vi "GetEventFrameInformation.vi"(8 "error in (no error)":errorcluster, 11 "Device Ref in":T3 format="%.0x") -> (0 "error out":errorcluster, 2 "EventFrames":T1[](array[typedef]) {"Channel Data Ref" format="%.0x"}, 3 "Device Ref out":T3 format="%.0x")   [LabVIEW 2020, in "FlexRay Custom Device Engine.lvlib"]
uses:
  FlexRay Custom Device Engine.lvlib
  <vilib>/NI VeriStand/Custom Device API/Custom Device Item Ref.ctl
  Shared/FREventInfo.ctl
  <vilib>/NI VeriStand/Custom Device API/Data Reference.ctl
  <vilib>/NI VeriStand/Custom Device API/Data Access Type.ctl
  Shared/Constants.vi
  <vilib>/NI VeriStand/Custom Device API/Get Item Property (Variant).vi
  <vilib>/NI VeriStand/Custom Device API/Custom Device API.lvlib
  <vilib>/NI VeriStand/Custom Device Tools/Custom Device Utility Library/Custom Device Utility Library.lvlib
  Shared/FlexRay Custom Device Shared.lvlib
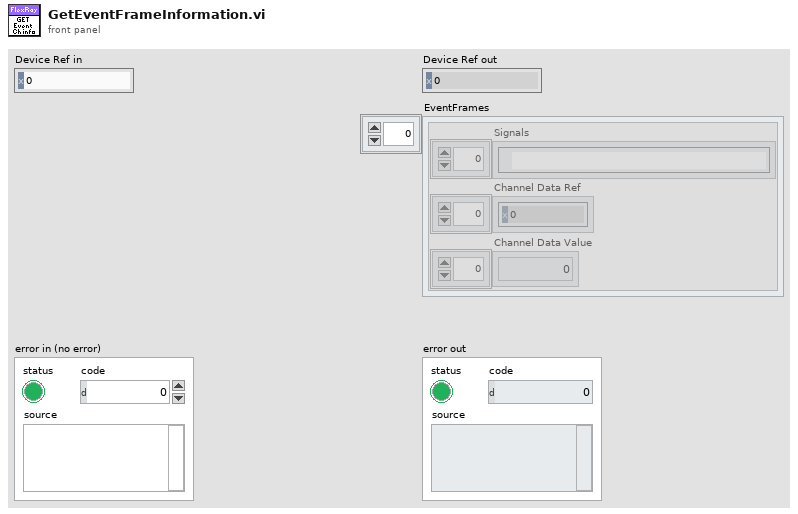
[diagram p1: front panel]
types:
  T1 = typedef "FlexRay Custom Device Shared.lvlib/FREventInfo.ctl" = cluster{"Signals":refnum<k21>[], "Channel Data Ref":T2[], "Channel Data Value":dbl[]}
  T2 = typedef "Custom Device API.lvlib/Data Reference.ctl" = i32
  T3 = typedef "Custom Device API.lvlib/Custom Device Item Ref.ctl" = u64
  T4 = typedef "Custom Device API.lvlib/Data Access Type.ctl" = enum16{"Read", "Write"}
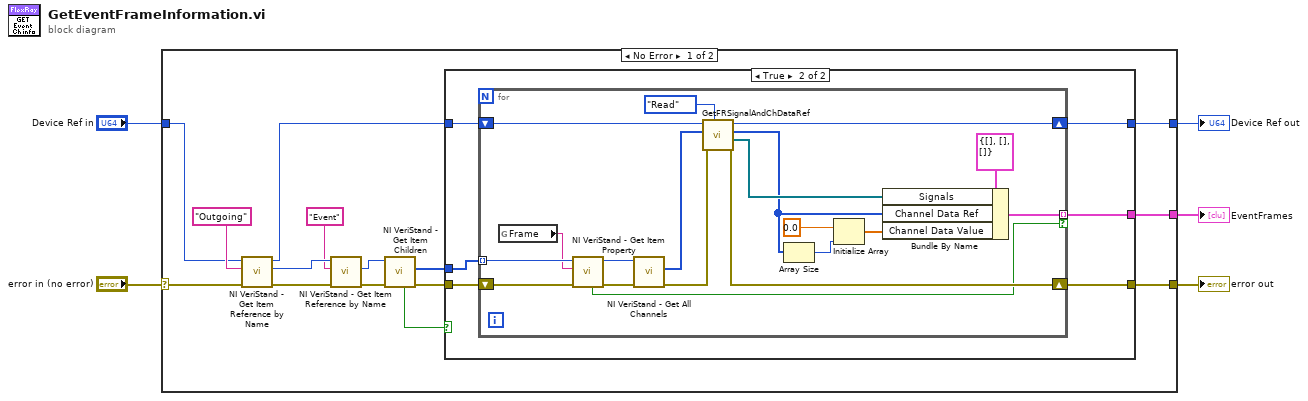
[diagram p0: block diagram]
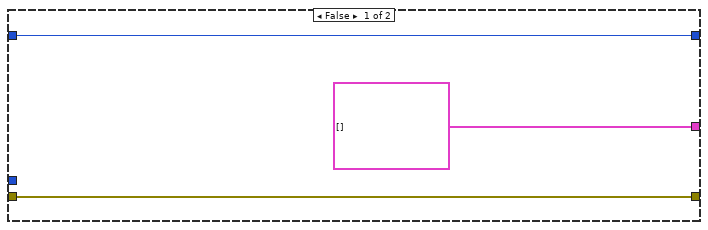
[diagram p2: hidden frame]
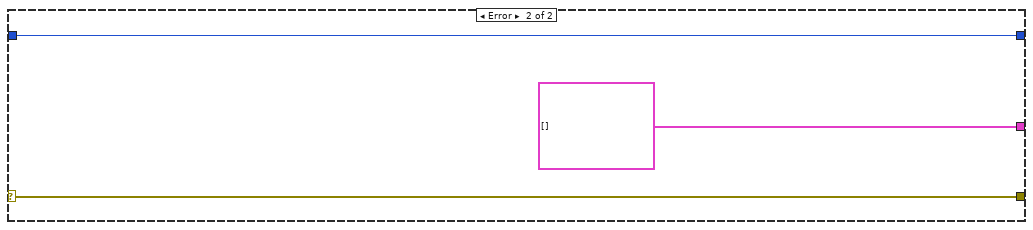
[diagram p3: hidden frame]
diagram:
  n1 = case shown="No Error" "error in (no error)" {
    selector: "error in (no error)" -> [w9 w50]
    tunnel: [w20 w50] -> w5
    tunnel: [w19 w51] -> w4
    tunnel: "Device Ref in" -> [w16 w51]
    tunnel: [w6 T1[] []] -> w1
    frame No Error {
      n2 = call <vilib>:"NI VeriStand - Get Item Reference by Name.vi"("error in (no error)"=w9, "Item Name"="Outgoing" ("Section Name"), "Parent Ref in"=w16) -> ("error out"=w15:errorcluster, "Item Ref"=w14:T3, "Parent Ref out"=w7:T3)  [unwired: 5 in, 1 out]
      n3 = call <vilib>:"NI VeriStand - Get Item Reference by Name.vi"("error in (no error)"=w15, "Item Name"="Event", "Parent Ref in"=w14) -> ("error out"=w13:errorcluster, "Item Ref"=w11:T3)  [unwired: 5 in, 2 out]
      n4 = call <vilib>:"NI VeriStand - Get Item Children.vi"("error in (no error)"=w13, "Item Ref in"=w11) -> ("error out"=w8:errorcluster, "Child Refs"=w18:T3[], "Found"=w10:bool)  [unwired: 6 in, 1 out]
      n5 = case shown="True" w10 {
        tunnel: w7 -> [w22 w29]
        tunnel: [w22 w28] -> w19
        tunnel: w8 -> [w23 w27]
        tunnel: [w23 w26] -> w20
        tunnel: w18 -> [_ w25]
        tunnel: [T1[] [] w24] -> w6
        frame False {
        }
        frame True {
          n6 = for {
            shift-right: [w43] -> w28
            shift-left: w29 -> [w46]
            shift-right: [w41] -> w26
            shift-left: w27 -> [w31]
            tunnel: w25 -> [w48] mode=indexing
            tunnel: [w38] -> w24 mode=indexing if=w33
            n7 = global read "Constants.vi" "Frame"() -> (w47:string)
            n8 = call-poly <vilib>:"NI VeriStand - Get Item Property.vi"("error in (no error)"=w31, "Property Name"=w47, "Item Ref in"=w48) -> ("error out"=w30:errorcluster, "Item Ref out"=w32:T3, "Found?"=w33:bool)  [unwired: 5 in, 1 out]
            n9 = call <vilib>:"NI VeriStand - Get All Channels.vi"("error in"=w30, "Section Ref in"=w32) -> ("error out"=w44:errorcluster, "Channel Refs"=w45:T3[])  [unwired: 6 in, 2 out]
            n10 = call "GetFRSignalAndChDataRef.vi"("Access"=Data_Access_Type."Read", "error in (no error)"=w44, "Channel Refs"=w45, "Device Ref in"=w46) -> ("error out"=w41:errorcluster, "FR Signals"=w39:refnum<k21>[], "Channel Data Ref"=w37:T2[], "Device Ref out"=w43:T3)  [unwired: 4 in]
            n11 = Array Size(array=w37) -> (size(s)=w35:i32)
            n12 = Initialize Array(0.0 ("element"), w35) -> (w36:dbl[])
            n13 = Bundle By Name(cluster=T1 {"Signals"=[], "Channel Data Ref"=[], "Channel Data Value"=[]} ("EventFrameChannelInfo"), "Signals"=w39, "Channel Data Ref"=w37, "Channel Data Value"=w36) -> (w38:T1)
          }
        }
      }
    }
    frame Error {
    }
  }
  "error out" <- w5
  "Device Ref out" <- w4
  "EventFrames" <- w1
